vi "Show Hardware parameters.vi"() -> ()   [LabVIEW 2023]
panel:
  in  "temp":dbl
  in  "VISA resource name":refnum<visa-resource-name>
  out "Ram Percentage":dbl(slide) scale=0.0..100.0
  out "GPU Temp":dbl
  out "CPU Percentage":dbl
  out "CPU Cores":dbl
  out "CPU Percentage":dbl(knob) scale=0.0..100.0
  out "CPU Frequency":dbl(knob) scale=0.0..4000.0
  in  "stop":bool
  out "GPU Temp":dbl(slide) scale=0.0..100.0
  in  "module path":path
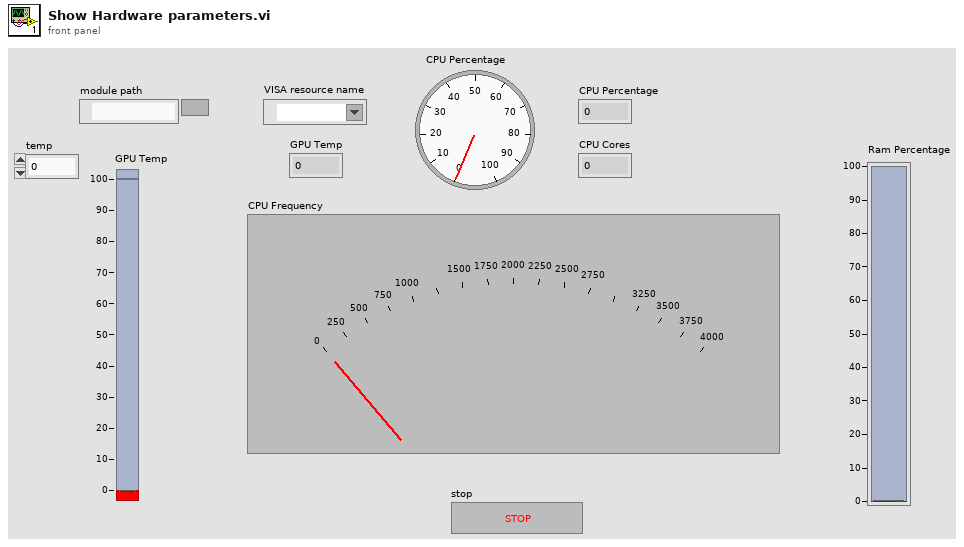
[diagram p1: front panel]
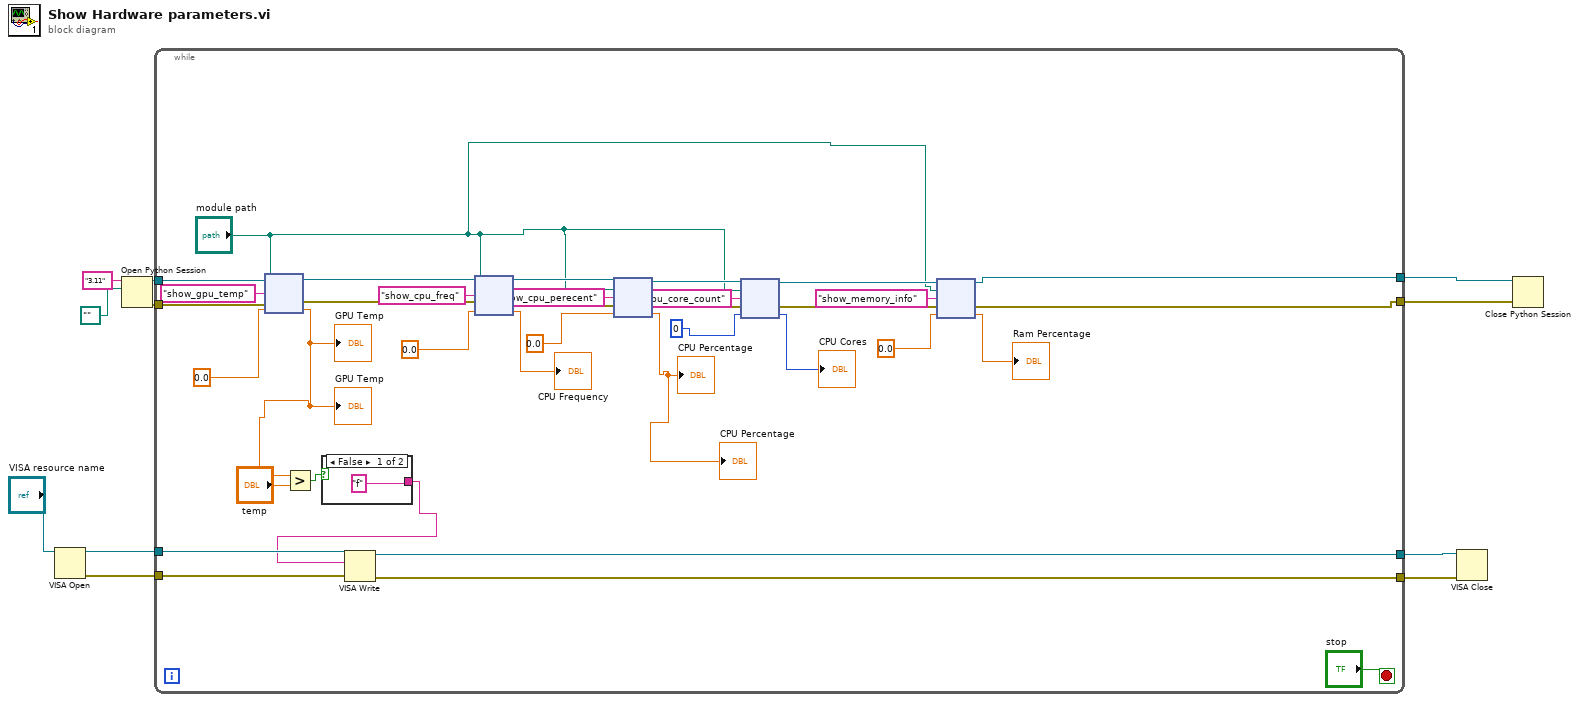
[diagram p0: block diagram]
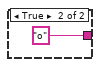
[diagram p2: hidden frame]
diagram:
  n1 = VISA Open(VISA resource name="VISA resource name") -> (VISA resource name=w4:refnum<visa-resource-name>, error out=w3:errorcluster)  [unwired: 4 in]
  n2 = Open Python Session(python version="3.11" ("Python version"), python path=path "" ("Python path")) -> (session out=w9:refnum<k35>, error out=w8:errorcluster)  [unwired: 1 in]
  n3 = while {
    tunnel: w9 -> [w47]
    tunnel: w8 -> [w46]
    tunnel: [w23] -> w7
    tunnel: [w22] -> w6
    tunnel: w4 -> [w19]
    tunnel: w3 -> [w18]
    tunnel: [w17] -> w2
    tunnel: [w16] -> w1
    stop <- "stop" stop-if-true
    n4 = node(w47, "module path", "show_gpu_temp" ("function name"), w46, 0.0) -> (w42:refnum<k35>, w41:errorcluster, w15:dbl)  [unwired: 2 out]
    "GPU Temp" <- w15
    "GPU Temp" <- w15
    n5 = Greater?(x=w15, y="temp") -> (0:w14:bool)
    n6 = case shown="False" w14 {
      tunnel: ["f" "o"] -> w13
      frame False {
      }
      frame True {
      }
    }
    n7 = VISA Write(VISA resource name=w19, write buffer=w13, error in (no error)=w18) -> (VISA resource name out=w17:refnum<visa-resource-name>, error out=w16:errorcluster)  [unwired: 1 out]
    n8 = node(w42, "module path", "show_cpu_freq" ("function name"), w41, 0.0) -> (w37:refnum<k35>, w36:errorcluster, →"CPU Frequency":dbl)  [unwired: 2 out]
    n9 = node(w37, "module path", "show_cpu_perecent" ("function name"), w36, 0.0) -> (w34:refnum<k35>, w33:errorcluster, →"CPU Percentage" →"CPU Percentage":dbl)  [unwired: 2 out]
    n10 = node(w34, "module path", "cpu_core_count" ("function name"), w33, 0) -> (w27:refnum<k35>, w26:errorcluster, →"CPU Cores":i32)  [unwired: 2 out]
    n11 = node(w27, "module path", "show_memory_info" ("function name"), w26, 0.0) -> (w23:refnum<k35>, w22:errorcluster, →"Ram Percentage":dbl)  [unwired: 2 out]
  }
  n12 = VISA Close(VISA resource name=w2, error in (no error)=w1) -> ()  [unwired: 1 out]
  n13 = Close Python Session(session in=w7, error in=w6) -> ()  [unwired: 1 out]
